vi "CV Message Loop.vi"(8 "Error In":errorcluster, 9 "Data Notifier":refnum<notifier>, 10 "Data Queue":refnum<queue>, 11 "Message Queues":T1) -> (0 "Error Out":errorcluster)   [LabVIEW 2015, in "CV.lvlib"]
uses:
  CV.lvlib
  support VIs/Message Queue/All Message Queues.ctl
  support VIs/Message Queue/Message Cluster.ctl
  Hardware libraries/Hardware_Configuration.ctl
  CV Acquisition State.ctl
  <vilib>/Utility/error.llb/Error Cluster From Error Code.vi
  <vilib>/ErrorRing/Error Ring.xnode
  support VIs/Message Queue/Message Queue.lvlib
  Acquisition/Acquisition.lvlib
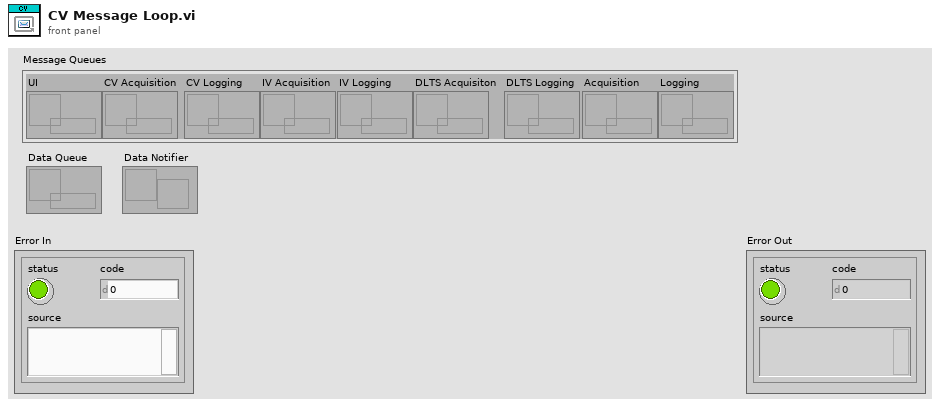
[diagram p1: front panel]
types:
  T1 = typedef "Message Queue.lvlib/All Message Queues.ctl" = cluster{"UI":refnum<queue>, "CV Acquisition":refnum<queue>, "CV Logging":refnum<queue>, "IV Acquisition":refnum<queue>, "IV Logging":refnum<queue>, "DLTS Acquisiton":refnum<queue>, "DLTS Logging":refnum<queue>, "Acquisition":refnum<queue>, "Logging":refnum<queue>}
  T2 = typedef "CV.lvlib/CV Acquisition State.ctl" = enum16{"Idle", "Acquiring"}
  T3 = typedef "Hardware_Configuration.ctl" = cluster{"Capacitance Meter":string, "Voltage Generator":string, "Pulse Generator":string, "Temperature Controller":string}
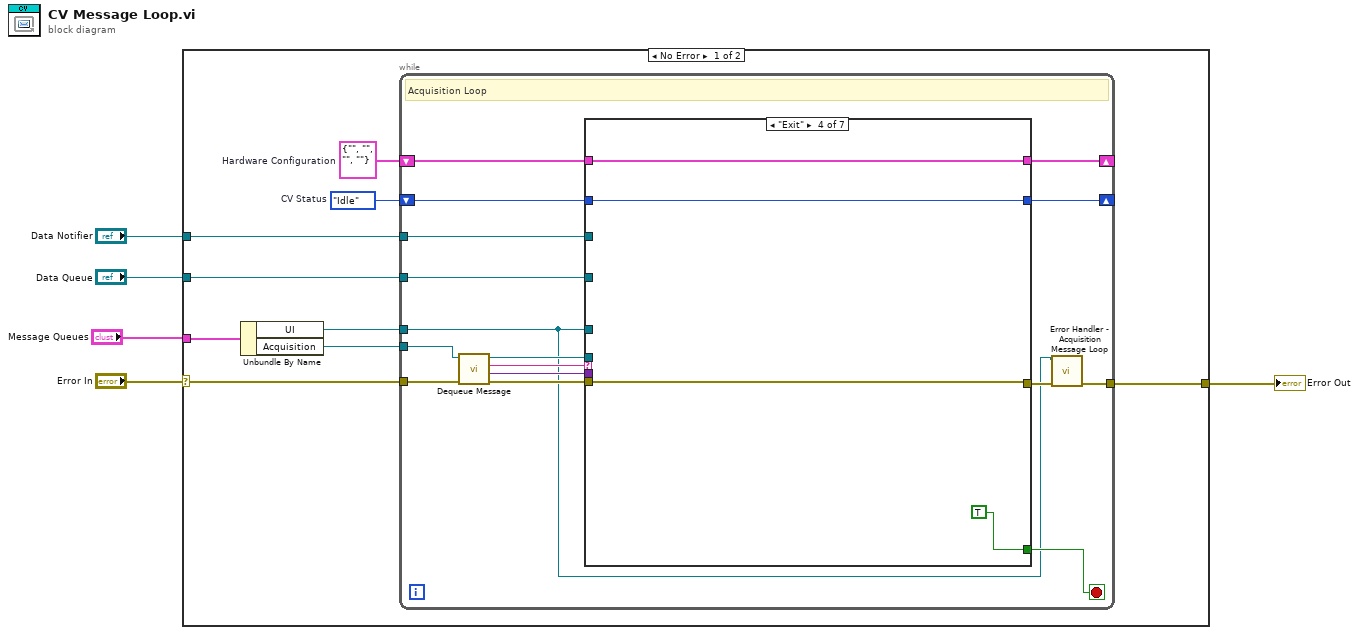
[diagram p0: block diagram]
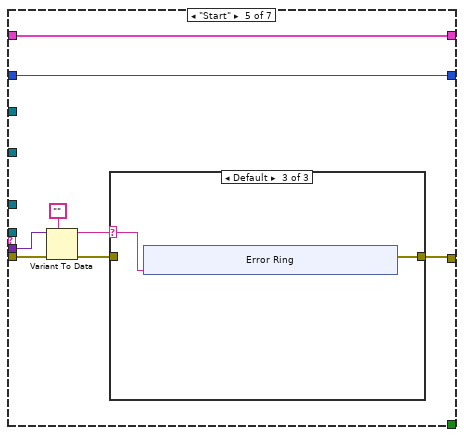
[diagram p5: hidden frame]
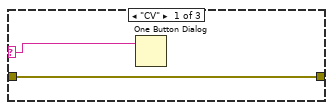
[diagram p6: hidden frame]
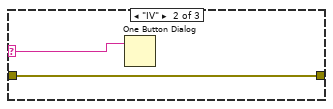
[diagram p7: hidden frame]
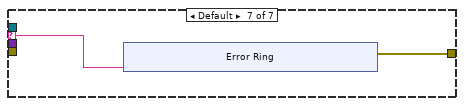
[diagram p10: hidden frame]
diagram:
  n1 = case shown="No Error" "Error In" {
    selector: "Error In" -> [w11 w83]
    tunnel: [w10 w83] -> w4
    tunnel: "Message Queues" -> [w14 _]
    tunnel: "Data Notifier" -> [w9 _]
    tunnel: "Data Queue" -> [w8 _]
    frame No Error {
      w6 = CV_Acquisition_State."Idle"  # CV Status
      w7 = T3 {"Capacitance Meter"="", "Voltage Generator"="", "Pulse Generator"="", "Temperature Controller"=""}  # Hardware Configuration
      n2 = Unbundle By Name(w14) -> ("UI"=w13:refnum<queue>, "Acquisition"=w12:refnum<queue>)
      n3 = while {
        tunnel: w13 -> [w15]
        tunnel: w12 -> [w30]
        tunnel: w11 -> [w26]
        tunnel: [w17] -> w10
        tunnel: w9 -> [w24]
        tunnel: w8 -> [w25]
        shift-right: [w22] -> _
        shift-left: w6 -> [w23]
        shift-right: [w21] -> _
        shift-left: w7 -> [w20]
        stop <- w19 stop-if-true
        # "Acquisition Loop"
        n4 = call "Dequeue Message.vi"("error in (no error)"=w26, "Message Queue"=w30) -> ("error out"=w27:errorcluster, "Message Data"=w28:variant, "Message"=w29:string, "dup Message Queue"=w16:refnum<queue>)  [unwired: 6 in]
        n5 = case shown="\"Exit\"" w29 {
          selector: w29 -> [_ _ _ _ _ _ w75]
          tunnel: w16 -> [_ _ _ _ _ w69 _]
          tunnel: w28 -> [_ _ _ _ w49 _ _]
          tunnel: w27 -> [w32 w35 w38 w42 w48 w66 _]
          tunnel: [w32 w35 w38 w42 w46 w65 w74] -> w18
          tunnel: w25 -> [_ _ _ _ _ w68 _]
          tunnel: w24 -> [_ _ _ _ _ w67 _]
          tunnel: w23 -> [w31 w34 w37 w41 w50 w71 _]
          tunnel: [w31 w34 w37 w41 w50 w70 _] -> w22
          tunnel: [w33 w36 w39 w43 w51 _ _] -> w21
          tunnel: w20 -> [w33 w36 w39 w43 w51 _ _]
          tunnel: [_ _ _ TRUE _ _ _] -> w19
          tunnel: w15 -> [_ _ _ _ _ _ _]
          frame "Initialize" {
          }
          frame "Stop" {
          }
          frame "Update Settings" {
          }
          frame "Exit" {
          }
          frame "Start" {
            n6 = Variant To Data(error in=w48, type="", Variant=w49) -> (data=w45:string, error out=w47:errorcluster)
            n7 = case shown="Default" w45 {
              selector: w45 -> [w52 w54 w56]
              tunnel: w47 -> [w53 w55 _]
              tunnel: [w53 w55 w57] -> w46
              frame "CV" {
                n8 = One Button Dialog(message=w52) -> ()  [unwired: 1 in, 1 out]
              }
              frame "IV" {
                n9 = One Button Dialog(message=w54) -> ()  [unwired: 1 in, 1 out]
              }
              frame Default {
                n10 = xnode "Error Ring"("parameter 0"=w56) -> ("error out"=w57:errorcluster)
              }
            }
          }
          frame "Acquire" {
            n11 = case shown="\"Acquiring\"" w71 {
              selector: w71 -> [_ w73]
              tunnel: [_ w73] -> w70
              tunnel: w69 -> [_ _]
              tunnel: w68 -> [_ _]
              tunnel: w67 -> [_ _]
              tunnel: w66 -> [_ w72]
              tunnel: [_ w72] -> w65
              frame "Idle", Default {
              }
              frame "Acquiring" {
              }
            }
          }
          frame Default {
            n12 = xnode "Error Ring"("parameter 0"=w75) -> ("error out"=w74:errorcluster)
          }
        }
        n13 = call "Error Handler - Acquisition Message Loop.vi"("error in (no error)"=w18, "Message Queue"=w15) -> ("dup error in"=w17:errorcluster)  [unwired: 8 in, 1 out]
      }
    }
    frame Error {
    }
  }
  "Error Out" <- w4
